vi "GetLineage.vi"(8 "error in (no error)":errorcluster, 11 "SMO in":refnum<class "SMO.lvclass">) -> (0 "error out":errorcluster, 2 "Lineage":string[](array[string]), 3 "SMO out":refnum<class "SMO.lvclass">)   [LabVIEW 2019, in "SMO.lvclass"]
doc: "JKI State Machine Objects (SMO) 1.3.0.56\nJKI - JKI\nCopyright (c) 2017, JKI"
uses:
  SMO.lvclass
  Support/Attribute.Owner/Attribute.Owner.lvclass
  Support/Attribute.Owner/Attribute.Owner.lvclass/Attribute.Owner.ctl
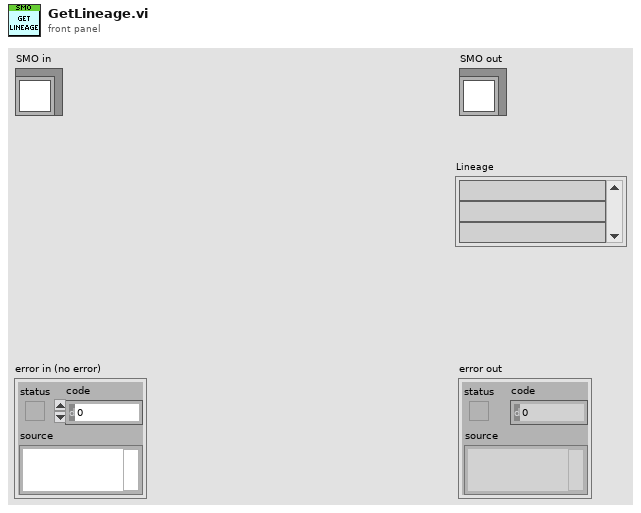
[diagram p1: front panel]
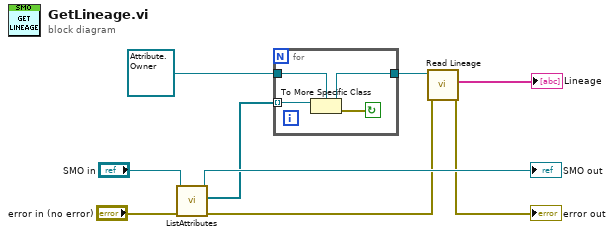
[diagram p0: block diagram]
diagram:
  n1 = call "ListAttributes.vi"("error in (no error)"="error in (no error)", "SMO in"="SMO in") -> ("error out"=w2:errorcluster, "[Attributes]"=w6:refnum<class "Attribute.lvclass">[], "SMO out"=→"SMO out":refnum<class "SMO.lvclass">)  [unwired: 7 in]
  n2 = for {
    tunnel: w6 -> [w13] mode=indexing
    tunnel: refnum<class "Attribute.Owner.lvclass"> refnum ("Attribute.Owner.lvclass") -> [w12]
    tunnel: [w10] -> w4
    stop <- w11 continue-if-true
    n3 = To More Specific Class(target class=w12, reference=w13) -> (specific class reference=w10:refnum<class "Attribute.Owner.lvclass">, error out=w11:errorcluster)  [unwired: 1 in]
  }
  n4 = call "Read Lineage.vi"("error in (no error)"=w2, "Attribute.Owner in"=w4) -> ("error out"=→"error out":errorcluster, "Lineage"=→"Lineage":string[])  [unwired: 7 in, 1 out]
